vi "Converting Temperatures.vi"() -> ()   [LabVIEW 2014]
panel:
  in  "Converting Fahrenheit to Celsius or Kelvin?":bool
  in  "Starting Temperature (C to K)":dbl
  in  "Starting Temperature (C to F)":dbl
  in  "Converting Celsius to Kelvin or Fahrenheit?":bool
  out "Converted Temperature 2":dbl(slide) scale=0.0..500.0
  in  "Starting Temperature (F to C)":dbl
  in  "Starting Temperature (F to K)":dbl
  out "Converted Temperature":dbl(slide) scale=0.0..1000.0
  # "Converting Temperature: K always false, C or F true"
  # "Starting Temperature: F=true, C=false"
  # "Celsius"
  # "Kelvin"
  # "Kelvin"
  # "Fahrenheit"
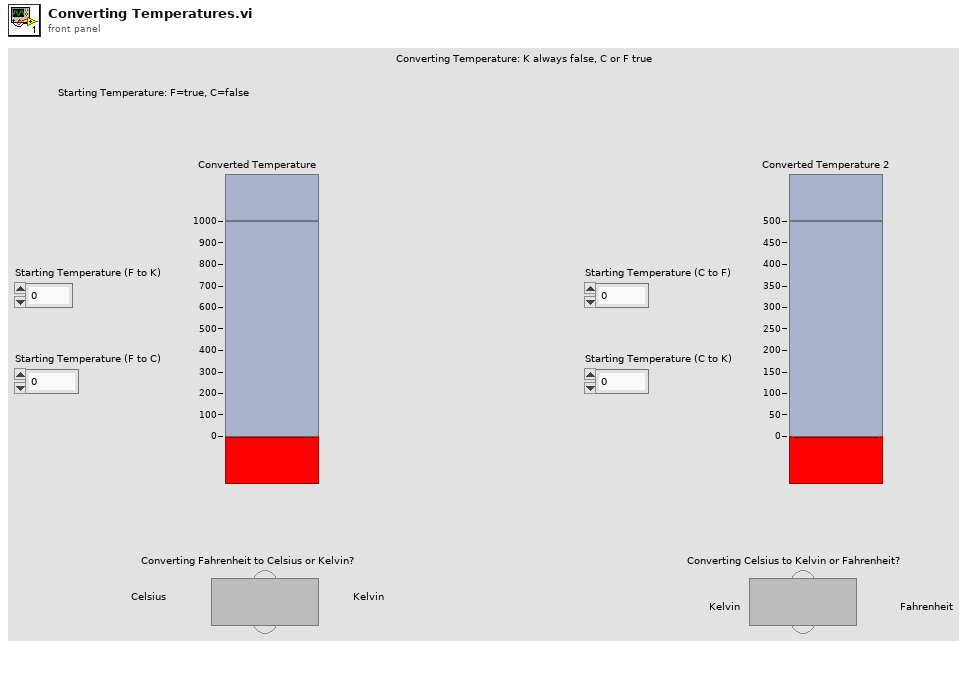
[diagram p1: front panel]
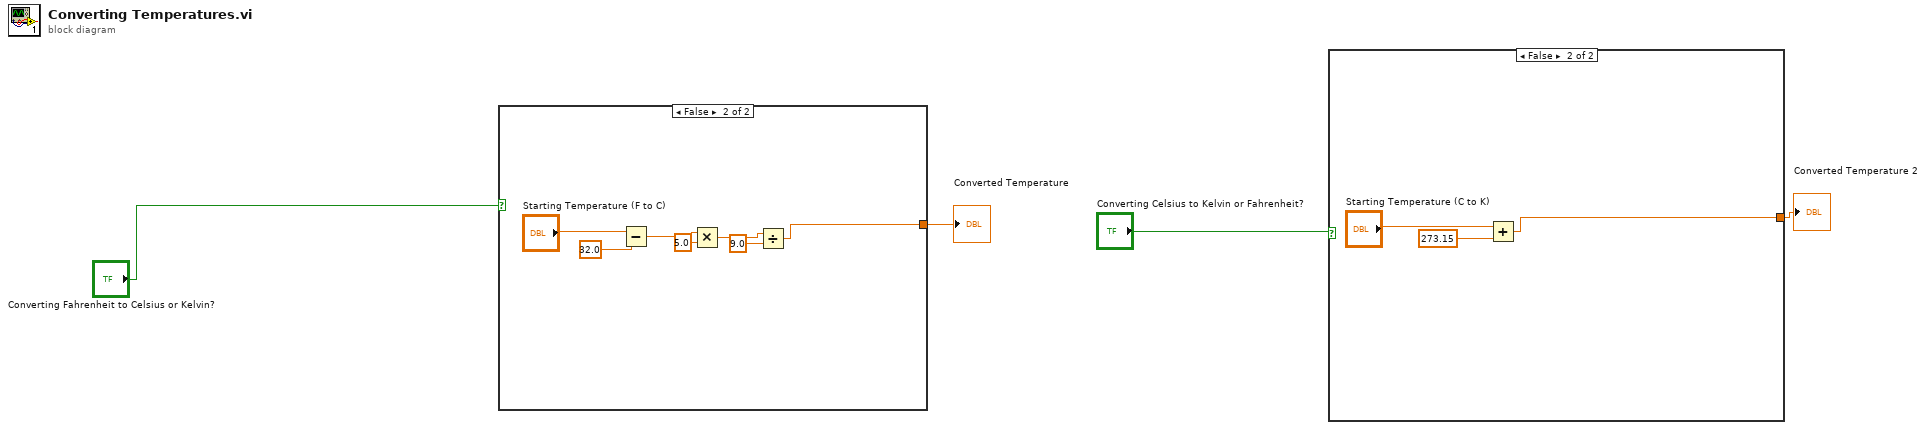
[diagram p0: block diagram]
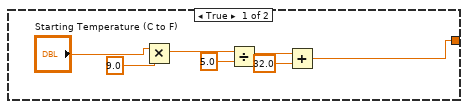
[diagram p2: hidden frame]
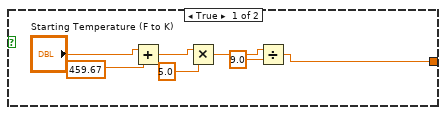
[diagram p3: hidden frame]
diagram:
  n1 = case shown="False" "Converting Fahrenheit to Celsius or Kelvin?" {
    tunnel: [w5 w12] -> w4
    frame True {
      n2 = Add(x="Starting Temperature (F to K)", y=459.67) -> (x+y=w9:dbl)
      n3 = Multiply(x=w9, y=5.0) -> (x*y=w7:dbl)
      n4 = Divide(x=w7, y=9.0) -> (x/y=w5:dbl)
    }
    frame False {
      n5 = Subtract(x="Starting Temperature (F to C)", y=32.0) -> (x-y=w16:dbl)
      n6 = Multiply(x=w16, y=5.0) -> (x*y=w14:dbl)
      n7 = Divide(x=w14, y=9.0) -> (x/y=w12:dbl)
    }
  }
  "Converted Temperature" <- w4
  n8 = case shown="False" "Converting Celsius to Kelvin or Fahrenheit?" {
    tunnel: [w19 w26] -> w2
    frame True {
      n9 = Multiply(x="Starting Temperature (C to F)", y=9.0) -> (x*y=w23:dbl)
      n10 = Divide(x=w23, y=5.0) -> (x/y=w21:dbl)
      n11 = Add(x=w21, y=32.0) -> (x+y=w19:dbl)
    }
    frame False {
      n12 = Add(x="Starting Temperature (C to K)", y=273.15) -> (x+y=w26:dbl)
    }
  }
  "Converted Temperature 2" <- w2
